vi "xy-chart (SubVI).vi"(8 "Draw Lissajous":bool, 10 "Signal 2":dbl, 11 "Signal 1":dbl) -> (3 "XY Graph 2":cluster{dbl[], dbl[]}(graph))   [LabVIEW 2021]
panel:
  out "size(s)":i32
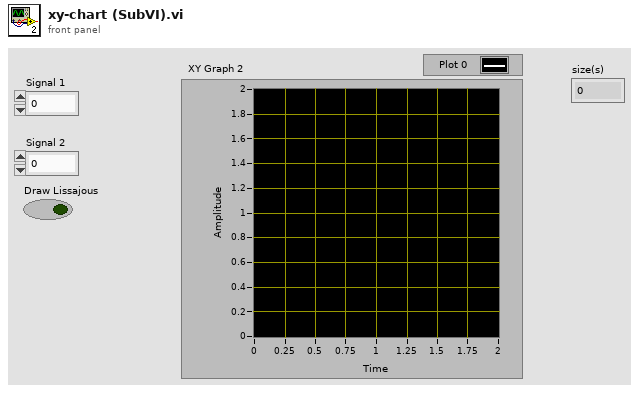
[diagram p1: front panel]
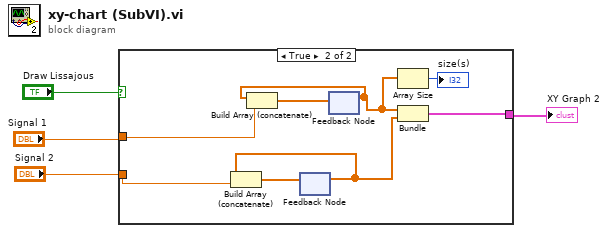
[diagram p0: block diagram]
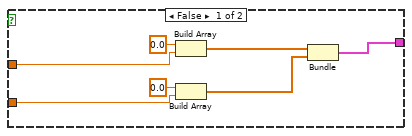
[diagram p2: hidden frame]
diagram:
  n1 = case shown="True" "Draw Lissajous" {
    tunnel: "Signal 2" -> [w6 w18]
    tunnel: "Signal 1" -> [w10 w17]
    tunnel: [w9 w15] -> w2
    frame False {
      n2 = Build Array(0.0 ("array"), w10) -> (w8:dbl[])
      n3 = Build Array(0.0 ("array"), w6) -> (w5:dbl[])
      n4 = Bundle(w8, w5) -> (w9:cluster{dbl[], dbl[]})  [unwired: 1 in]
    }
    frame True {
      n5 = feedback #1() -> (w19:dbl[])  [unwired: 1 in]
      n6 = Build Array (concatenate)(w19, w18) -> (w16:dbl[])
      n7 = feedback-in #1(w16) -> ()
      n8 = feedback #2() -> (w13:dbl[])  [unwired: 1 in]
      n9 = Build Array (concatenate)(w13, w17) -> (w14:dbl[])
      n10 = feedback-in #2(w14) -> ()
      n11 = Array Size(array=w13) -> (size(s)=→"size(s)":i32)
      n12 = Bundle(w13, w19) -> (w15:cluster{dbl[], dbl[]})  [unwired: 1 in]
    }
  }
  "XY Graph 2" <- w2
